vi "Clean Targets.vi"(0 "Targets In":T1[](array[typedef]), 1 "error in":errorcluster) -> (2 "Problems":bool, 3 "Targets Out":T1[](array[typedef]), 4 "error out":errorcluster)   [LabVIEW 2013]
uses:
  Data Access Objects/Application/Number Of LBCBs.ctl
  Data Access Objects/Metadata/LBCB Number.ctl
  Data Access Objects/Metadata/Persistant DAO Actions.ctl
  MixedMode/Messages/Target.ctl
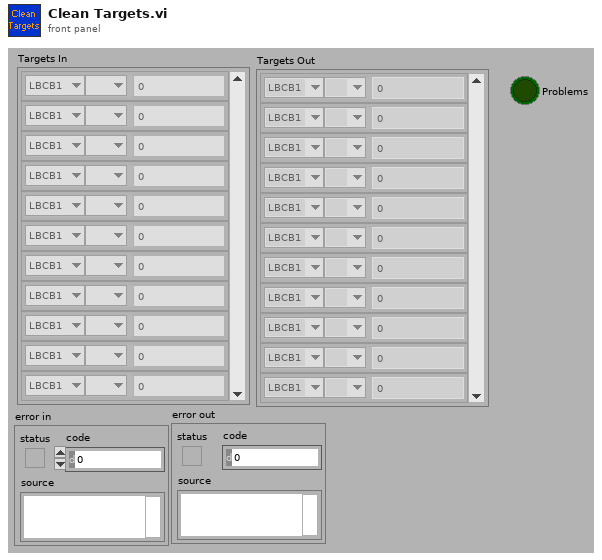
[diagram p1: front panel]
types:
  T1 = typedef "Target.ctl" = cluster{"LBCB Number":T2, "DOF Vectors":enum16{" ", "Dx", "Dy", "Dz", "Rx", "Ry", "Rz", "Fx", "Fy", "Fz", "Mx", "My", "Mz"}, "Amount":dbl}
  T2 = typedef "LBCB Number.ctl" = enum16{"LBCB1", "LBCB2"}
  T3 = typedef "Persistant DAO Actions.ctl" = enum16{"Init", "Get", "Set", "Load", "Save"}
  T4 = typedef "Number Of LBCBs.ctl" = enum16{"1", "2"}
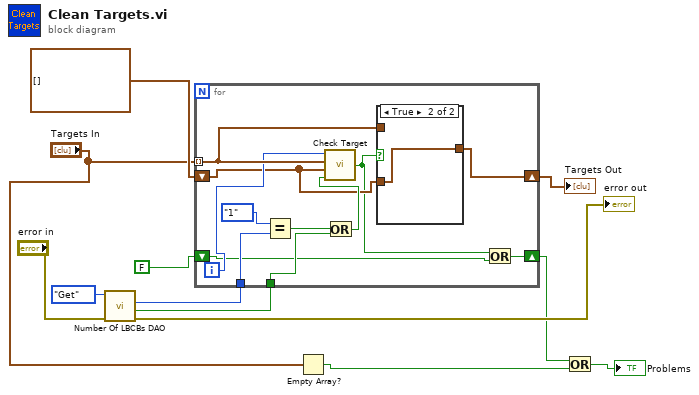
[diagram p0: block diagram]
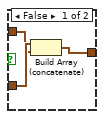
[diagram p2: hidden frame]
diagram:
  n1 = call "Number Of LBCBs DAO.vi"("error in (no error)"="error in", "Actions"=Persistant_DAO_Actions."Get") -> ("error out"=→"error out":errorcluster, "Rigid Connection Out"=w8:bool, "Number of\nLBCBs Out"=w7:T4)  [unwired: 6 in, 1 out]
  n2 = for {
    tunnel: "Targets In" -> [w19] mode=indexing
    tunnel: w7 -> [w24]
    tunnel: w8 -> [w21]
    shift-right: [w18] -> w11
    shift-left: T1[] [] -> [w16]
    shift-right: [w15] -> w2
    shift-left: FALSE ("Problems") -> [w13]
    i -> [w17]
    n3 = Equal?(x=Number_Of_LBCBs."1", y=w24) -> (x = y?=w22:bool)
    n4 = Or(x=w22, y=w21) -> (x .or. y?=w20:bool)
    n5 = call "Check Target.vi"("Is 1 LBCB"=w20, "Other Targets"=w16, "Target"=w19, "Index"=w17) -> ("Problems"=w14:bool)
    n6 = case shown="True" w14 {
      tunnel: w16 -> [w27 w28]
      tunnel: w19 -> [w26 _]
      tunnel: [w25 w28] -> w18
      frame False {
        n7 = Build Array (concatenate)(w27, w26) -> (w25:T1[])
      }
      frame True {
      }
    }
    n8 = Or(x=w14, y=w13) -> (x .or. y?=w15:bool)
  }
  "Targets Out" <- w11
  n9 = Empty Array?(array="Targets In") -> (empty?=w1:bool)
  n10 = Or(x=w2, y=w1) -> (x .or. y?=→"Problems":bool)
